vi "Traverse-Main.vi"() -> ()   [LabVIEW 2017]
uses:
  TypeDefs/Trav-Command-TD.ctl
  Globals/Trav-Positon-Info.vi
  Settings/Traverse-Settings-Global.vi
panel:
  in  "Trav Command":T1 items=["Read Position", "Move"]
  in  "OK Button":bool
  in  "Z":dbl
  in  "Y":dbl
  in  "X":dbl
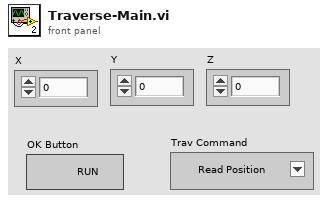
[diagram p1: front panel]
types:
  T1 = typedef "Trav-Command-TD.ctl" = u16
  T2 = typedef "Position-Info-TD.ctl" = cluster{"Current Position ABS":dbl[], "Current Position":dbl[], "Reference Position":dbl[], "Axis Names":string[]}
  T3 = typedef "Settings-Control.ctl" = cluster{"Acceleration":dbl[], "Deceleration":dbl[], "Max Velocity":dbl[], "Speed":dbl, "Pulse/Degree":dbl, "Degre Factor":dbl[], "mm/rotation":dbl[], "Traverse Name":string}
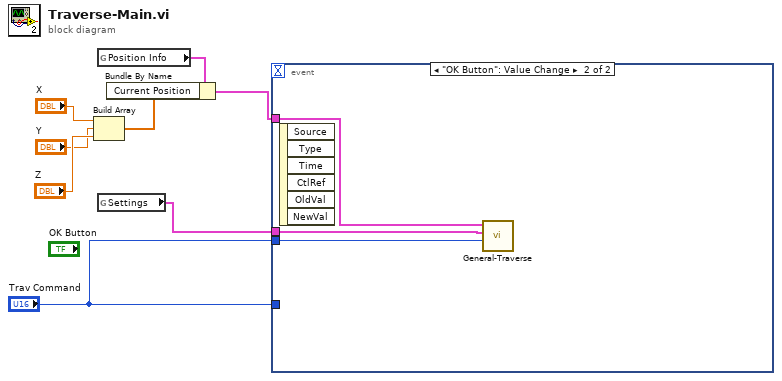
[diagram p0: block diagram]
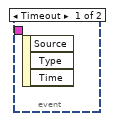
[diagram p2: hidden frame]
diagram:
  n1 = Build Array("X", "Y", "Z") -> (w4:dbl[])
  n2 = global read "Trav-Positon-Info.vi" "Position Info"() -> (w8:T2)
  n3 = global read "Traverse-Settings-Global.vi" "Settings"() -> (w2:T3)
  n4 = Bundle By Name(cluster=w8, "Current Position"=w4) -> (w3:T2)
  n5 = event shown="[1] \"OK Button\": Value Change" {
    selector: _ -> [_ _]
    dyn-events: _ -> [_ _]
    timeout: _ -> [_ _]
    tunnel: "Trav Command" -> [_ _]
    tunnel: "Trav Command" -> [_ w11]
    tunnel: w3 -> [_ w10]
    tunnel: w2 -> [_ w9]
    event Timeout {
      n6 = event-data() -> ()  [unwired: 1 in, 3 out]
    }
    event "OK Button": Value Change {
      n7 = event-data() -> ()  [unwired: 1 in, 6 out]
      n8 = call "General-Traverse.vi"("Trav Command"=w11, "Settings"=w9, "Position Info IN"=w10) -> ()  [unwired: 7 in, 2 out]
    }
  }
